vi "Galobal variable_TI.vi"() -> ()   [LabVIEW 2015]
uses:
  Control Button/Control 11.ctl
panel:
  out "Server":bool
  in  "Shift":T1
  out "Rework Bit":bool
  in  "NG Count":u8
  in  "Shift Change":string
  in  "OP":string
  in  "Feeder Empty":bool
  in  "LVDT Offset":T2=0.29 format="%0.03f"
  out "Led Enable RL v":bool
  out "Led Enable FR v":bool
  out "Led Enable FL v":bool
  out "Led Enable RR v":bool
  out "Led Enable RL":bool
  out "Led Enable FR":bool
  out "Led Enable FL":bool
  out "Led Enable RR":bool
  in  "LVDT Result bit":bool
  in  "OK /ng":i32
  in  "Channel":i32
  in  "Parameter":u8
  in  "RPT Bypass":bool
  in  "Clip Status":string
  in  "Height Status":string
  in  "Pokayoka Status":bool
  in  "Rpt Read":bool
  in  "Rpt Write":bool
  in  "DCNG":bool
  in  "DC OK":bool
  in  "LVDT Data":T3 {"LVDT4Max(mm) AI3" format="%0.02f"; "LVDT3Max(mm) AI2" format="%0.02f"; "LVDT2Max(mm) AI1" format="%0.02f"; "LVDT1Max(mm) AI0" format="%0.02f"; "LVDT4Min(mm) AI3" format="%0.02f"; "LVDT3Min(mm) AI2" format="%0.02f"; "LVDT2Min(mm) AI1" format="%0.02f"; "LVDT1Min (mm)AI0" format="%0.02f"}
  in  "Read LVDT Value":dbl[](array[numeric]) format="%0.03f"
  out "Result Lvdt":T4
  in  "Dist. data":dbl[](array[numeric]) format="%0.03f"
  in  "Color4":u32
  in  "Color3":u32
  in  "Color2":u32
  in  "Color1":u32
  in  "Ring Sensor Off  Bit":bool
  in  "Ring Sensor On Bit":bool
  in  "Desontter data 4":string
  in  "Desontter data 3":string
  in  "Desontter data 2":string
  in  "Desontter data1":string
  in  "Desontter data":i32
  out "AI_6212":bool[](array[boolean])
  in  "Job Id":string
  in  "LCD  Barcode_Trigger":bool
  in  "MIC Barcode _Trigger":bool
  in  "MIC Barcode":string="0UD6I20MUW7W"
  in  "LCD Barcode":string
  in  "Barcode Setting":T5={"MIC "="", "baud rate MIC "=9600, "LCD "="COM5", "baud rate_LCD"=115200}
  out "IL Sensor_Pokayoka":bool[](array[boolean])
  in  "Running Model":string
  in  "Sensor Setting Data":T6
  out "Sensor Data":T7
  in  "NI Comm.Error":bool
  in  "LVDT":dbl format="%0.03f"
  in  "Load Cell":dbl format="%0.03f"
  in  "Digital Output":bool[](array[boolean])
  in  "Auto Exit":bool
  in  "Slid Servo Home bit":bool
  in  "Call Home M2":bool
  in  "Call Home M1":bool
  in  "Barcode Lenght":i32
  in  "Barcode Scan Bit":bool
  in  "Barcode Data":string
  in  "Control Enable":bool
  in  "Stop M1":bool
  in  "Stop M2":bool
  in  "Programlist":string[](array[string])
  in  "STM Done Bit":bool
  in  "Offset_2":dbl
  in  "Offset_1":dbl
  in  "Slop _2":dbl
  in  "Slop_1":dbl
  out "Analoge Input":dbl[](array[numeric])
  out "AI_as DI":bool[](array[boolean])
  in  "Manual DO":bool[](array[boolean])
  in  "Manual CMD":bool
  out "File Path":path[](array[path])
  in  "Digital input":bool[](array[boolean])
  in  "User Name":string
  in  "Exit":bool
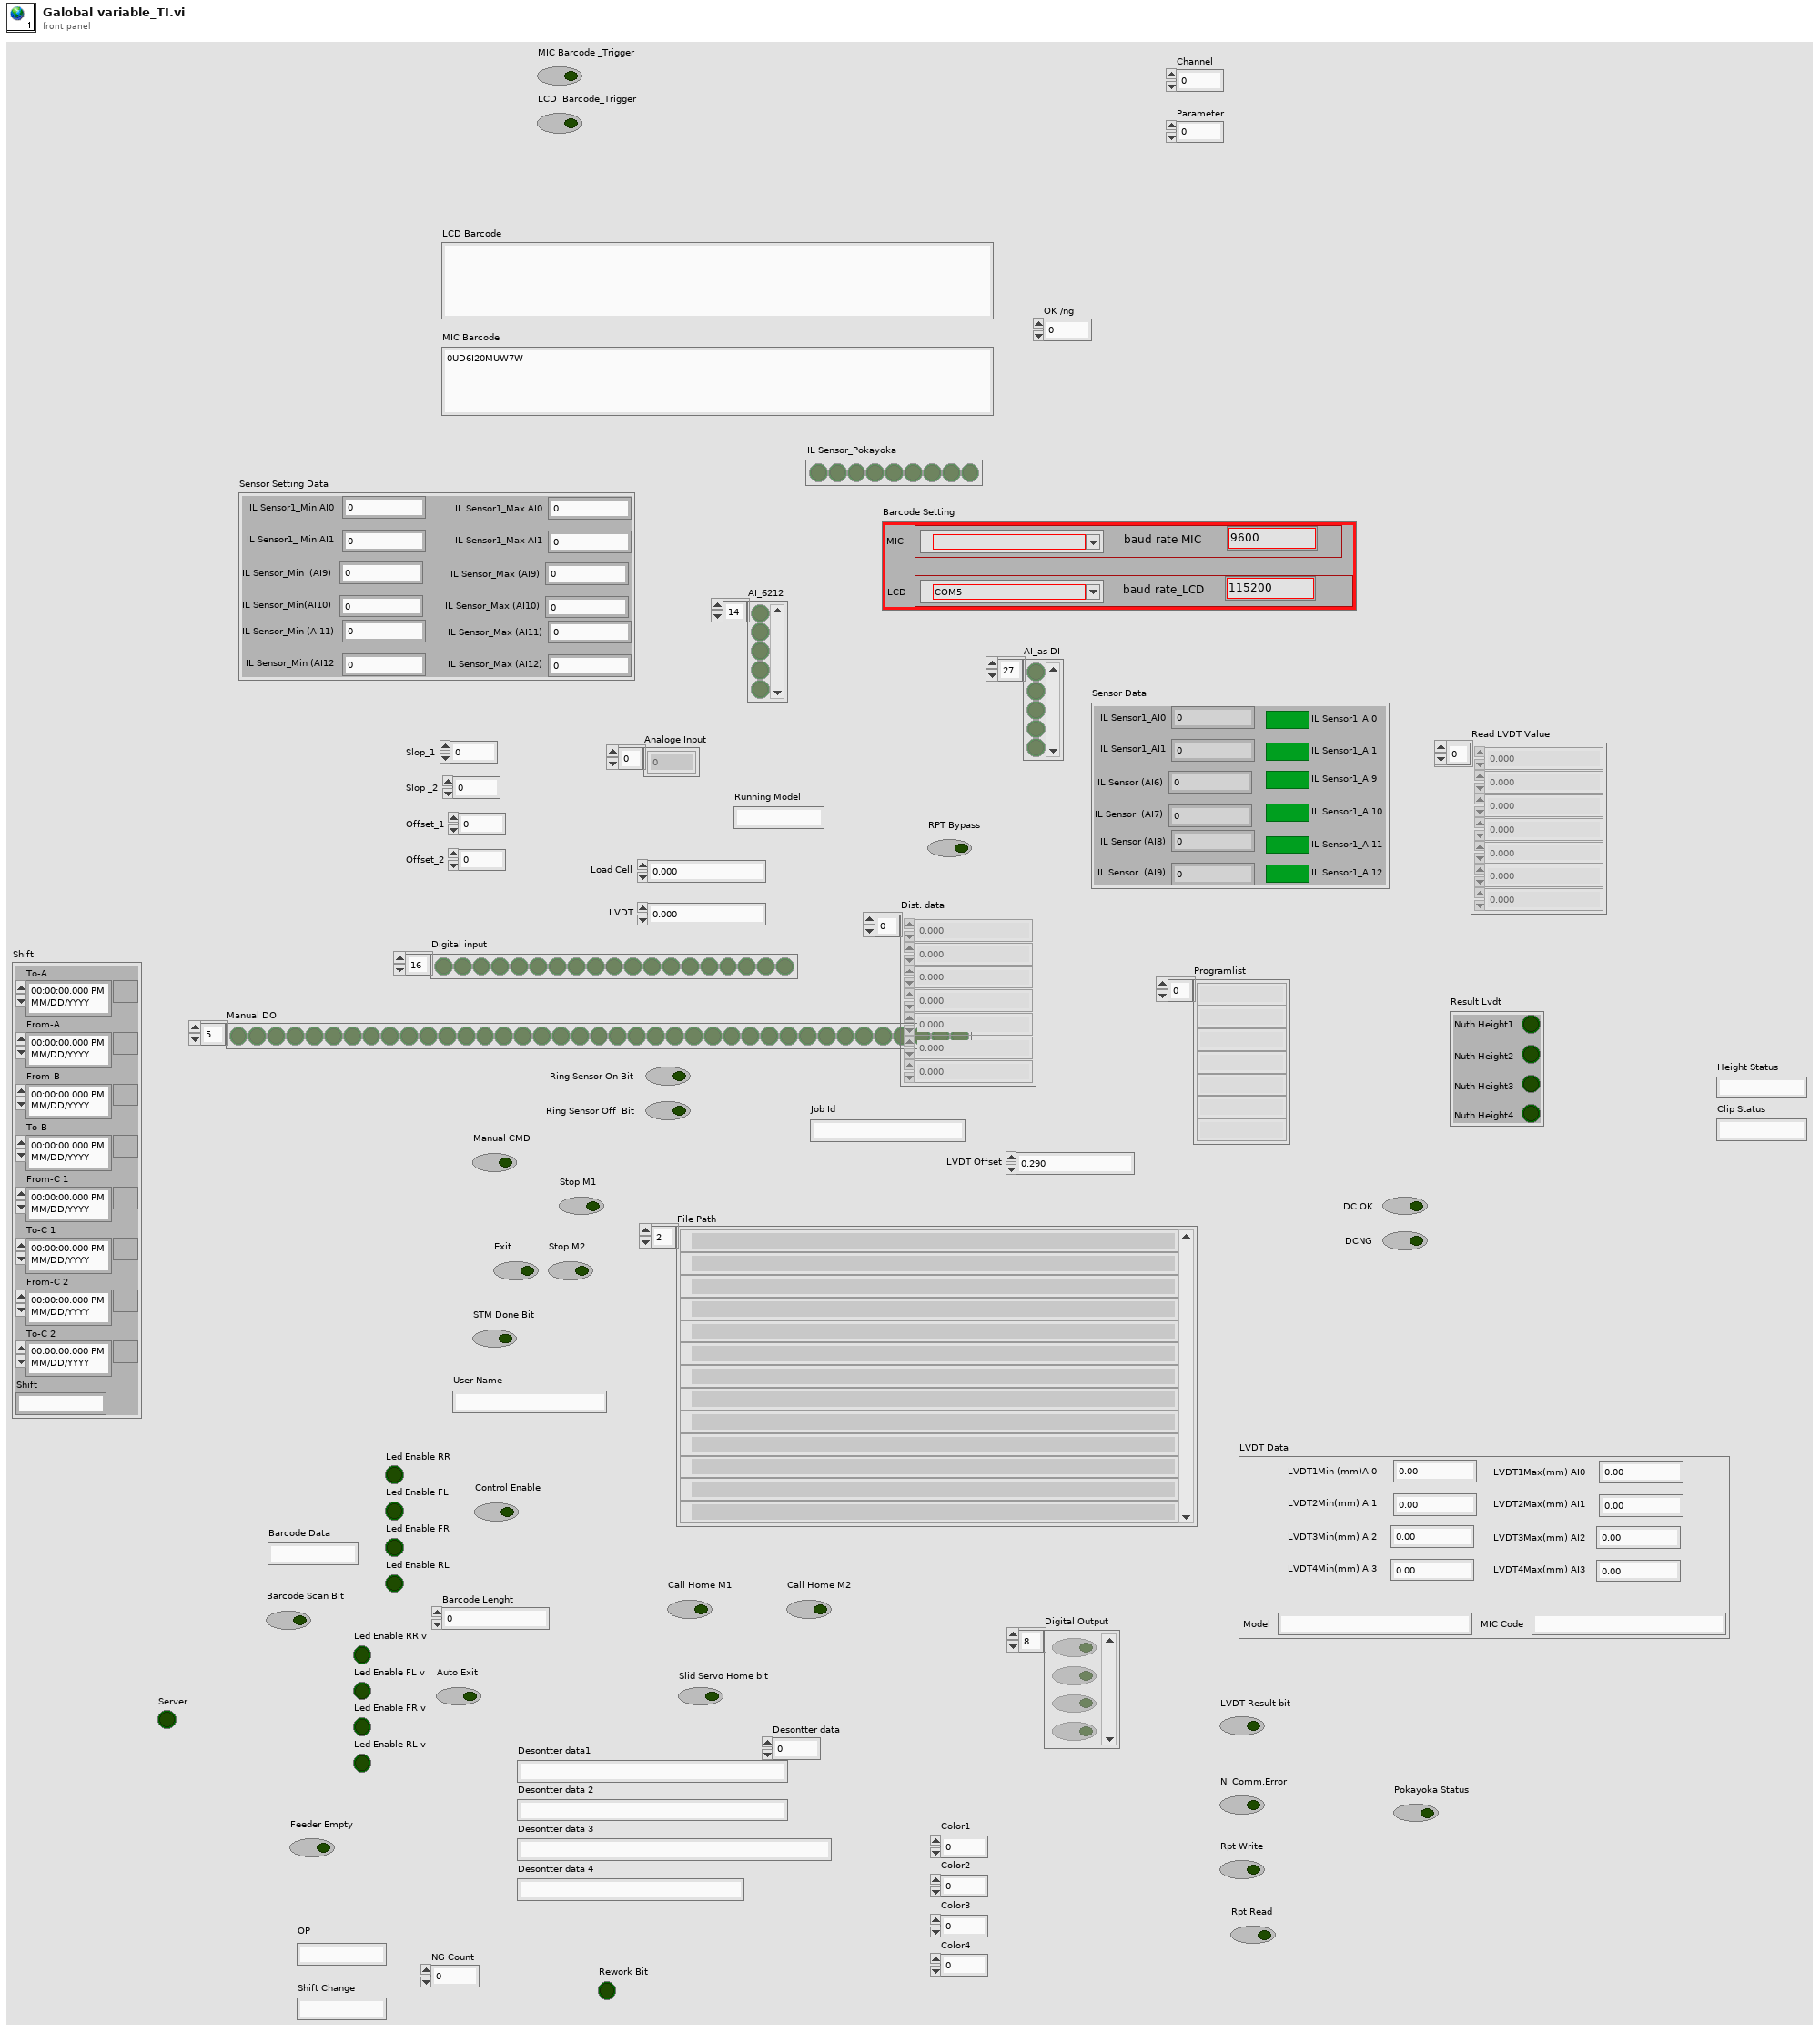
[diagram p1: front panel]
types:
  T1 = cluster{"To-A":timestamp, "From-A":timestamp, "From-B":timestamp, "To-B":timestamp, "From-C 1":timestamp, "To-C 1":timestamp, "From-C 2":timestamp, "To-C 2":timestamp, "Shift":string}
  T2 = typedef "Control 11.ctl" = dbl
  T3 = cluster{"LVDT1Max(mm) AI0":dbl, "LVDT1Min (mm)AI0":dbl, "LVDT2Max(mm) AI1":dbl, "LVDT2Min(mm) AI1":dbl, "LVDT3Max(mm) AI2":dbl, "LVDT3Min(mm) AI2":dbl, "LVDT4Max(mm) AI3":dbl, "LVDT4Min(mm) AI3":dbl, "Model":string, "MIC Code":string}
  T4 = cluster{"Nuth Height1":bool, "Nuth Height2":bool, "Nuth Height3":bool, "Nuth Height4":bool}
  T5 = cluster{"MIC ":refnum<visa-resource-name>, "baud rate MIC ":u32, "LCD ":refnum<visa-resource-name>, "baud rate_LCD":u32}
  T6 = cluster{"IL Sensor1_Max AI0":dbl, "IL Sensor1_Min AI0":dbl, "IL Sensor1_Max AI1":dbl, "IL Sensor1_ Min AI1":dbl, "IL Sensor_Max (AI9)":dbl, "IL Sensor_Min  (AI9)":dbl, "IL Sensor_Max (AI10)":dbl, "IL Sensor_Min(AI10)":dbl, "IL Sensor_Max (AI11)":dbl, "IL Sensor_Min (AI11)":dbl, "IL Sensor_Max (AI12)":dbl, "IL Sensor_Min (AI12":dbl}
  T7 = cluster{"IL Sensor1_AI0":dbl, "IL Sensor1_AI1":dbl, "IL Sensor (AI6)":dbl, "IL Sensor  (AI7)":dbl, "IL Sensor (AI8)":dbl, "IL Sensor  (AI9)":dbl, "IL Sensor1_AI0":bool, "IL Sensor1_AI1":bool, "IL Sensor1_AI9":bool, "IL Sensor1_AI10":bool, "IL Sensor1_AI11":bool, "IL Sensor1_AI12":bool}
diagram:
